vi "get next modbus address.vi"(0 "Modbus Slave configuration in":refnum<class "Modbus Slave configuration.lvclass">, 5 "modbus channels":refnum<class "Modbus Module Channel.lvclass">[](array[class]), 7 "modbus address":T1(array[cluster]), 9 "channel indices":i32[](array[numeric]), 11 "error in":errorcluster) -> (4 "Modbus Slave configuration out":refnum<class "Modbus Slave configuration.lvclass">, 8 "modbus address out":T1(array[cluster]), 15 "error out":errorcluster)   [LabVIEW 2013, in "Modbus Slave configuration.lvclass"]
uses:
  Modbus Slave configuration.lvclass
  module channel/Modbus Module Channel.lvclass
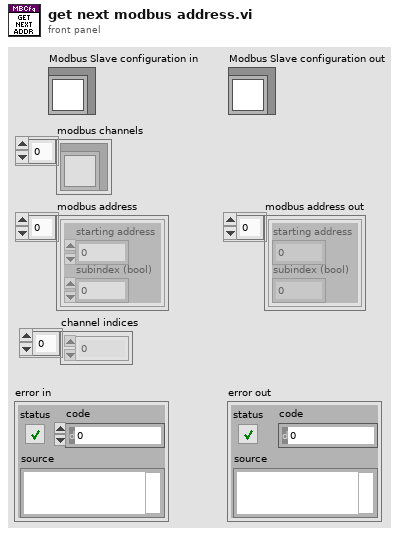
[diagram p1: front panel]
types:
  T1 = cluster{"starting address":u16, "subindex (bool)":i32}[]
  T2 = typedef "Modbus Module Channel.lvclass/data bank type.ctl" = enum16{"coils", "discrete inputs", "input registers", "holding registers"}
  T3 = typedef "tag bus.lvlib/tag descriptor.lvclass/Data Type.ctl" = enum16{"Double", "Single", "I64", "I32", "I16", "I8", "U64", "U32", "U16", "U8", "Boolean", "String", "Array of Double", "Array of Single", "Array of I64", "Array of I32", "Array of I16", "Array of I8", "Array of U64", "Array of U32", "Array of U16", "Array of U8", "Array of Boolean", "Array of String"}
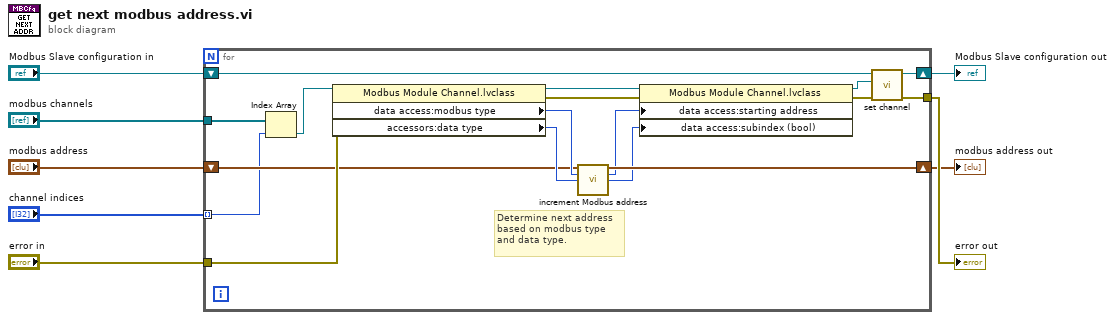
[diagram p0: block diagram]
diagram:
  n1 = for {
    tunnel: "modbus channels" -> [w10]
    shift-right: [w16] -> w1
    shift-left: "modbus address" -> [w17]
    shift-right: [w24] -> w5
    shift-left: "Modbus Slave configuration in" -> [w12]
    tunnel: "error in" -> [w23]
    tunnel: [w20] -> w6
    tunnel: "channel indices" -> [w11] mode=indexing
    # "Determine next address \nbased on modbus type \nand data type."
    n2 = Index Array(array=w10, index=w11) -> (element=w9:refnum<class "Modbus Module Channel.lvclass">)
    n3 = property class="Modbus Module Channel.lvclass"(reference=w9, error in=w23) -> (reference out=w13:refnum<class "Modbus Module Channel.lvclass">, error out=w22:errorcluster, "data access:modbus type"=w18:T2, "accessors:data type"=w19:T3)
    n4 = call "increment Modbus address.vi"("available addresses"=w17, "modbus type"=w18, "data type"=w19) -> ("available addresses out"=w16:T1, "starting address"=w15:u16, "subindex (bool)"=w14:i32)  [unwired: 10 in]
    n5 = property class="Modbus Module Channel.lvclass"(reference=w13, error in=w22, "data access:starting address"=w15, "data access:subindex (bool)"=w14) -> (reference out=w25:refnum<class "Modbus Module Channel.lvclass">, error out=w21:errorcluster)
    n6 = call "set channel.vi"("error in"=w21, "Modbus Module Channel.lvclass"=w25, "Modbus Slave configuration in"=w12) -> ("error out"=w20:errorcluster, "Modbus Slave configuration out"=w24:refnum<class "Modbus Slave configuration.lvclass">)  [unwired: 7 in]
  }
  "error out" <- w6
  "Modbus Slave configuration out" <- w5
  "modbus address out" <- w1
